vi "Day 12-1.vi"() -> ()   [LabVIEW 2020]
panel:
  out "# Paths 2":i32
  out "# Paths 1":i32
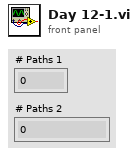
[diagram p1: front panel]
types:
  T1 = typedef "Cave System.ctl" = cluster{"Names":map{string, i32}, "Caves":T2[], "Start":i32, "End":i32}
  T2 = typedef "Cave.ctl" = cluster{"Name":string, "Index":i32, "Big":bool, "Links":i32[]}
  T3 = typedef "Path.ctl" = cluster{"Visited":bool[], "Caves":i32[]}
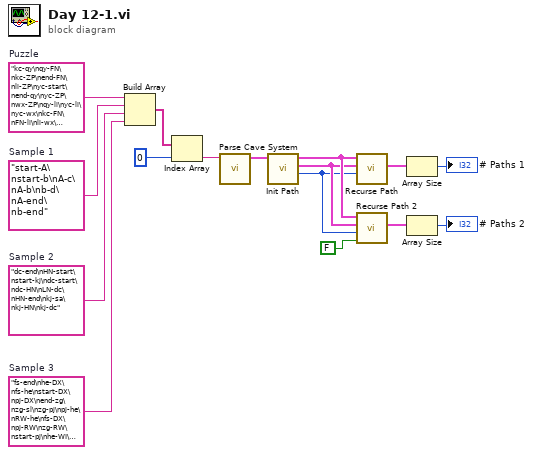
[diagram p0: block diagram]
diagram:
  w11 = "kc-qy\nqy-FN\nkc-ZP\nend-FN\nli-ZP\nyc-start\nend-qy\nyc-ZP\nwx-ZP\nqy-li\nyc-li\nyc-wx\nkc-FN\nFN-li\nli-wx\nkc-wx\nZP-start\nli-kc\nqy-nv\nZP-qy\nnv-xr\nwx-start\nend-nv\nkc-nv\nnv-XQ"  # Puzzle
  w14 = "fs-end\nhe-DX\nfs-he\nstart-DX\npj-DX\nend-zg\nzg-sl\nzg-pj\npj-he\nRW-he\nfs-DX\npj-RW\nzg-RW\nstart-pj\nhe-WI\nzg-he\npj-fs\nstart-RW"  # Sample 3
  w15 = "dc-end\nHN-start\nstart-kj\ndc-start\ndc-HN\nLN-dc\nHN-end\nkj-sa\nkj-HN\nkj-dc"  # Sample 2
  w16 = "start-A\nstart-b\nA-c\nA-b\nb-d\nA-end\nb-end"  # Sample 1
  n1 = Build Array(w11, w16, w15, w14) -> (w13:string[])
  n2 = Index Array(array=w13, index=0) -> (element=w10:string)
  n3 = call "Parse Cave System.vi"("Input"=w10) -> ("Cave System"=w9:T1)  [unwired: 10 in]
  n4 = call "Init Path.vi"("Cave System In"=w9) -> ("Start"=w4:i32, "Path"=w5:T3, "Cave System"=w6:T1)  [unwired: 8 in]
  n5 = call "Recurse Path.vi"("Next Cave"=w4, "Parent Path"=w5, "Cave System In"=w6) -> ("Found Paths"=w8:T3[])  [unwired: 8 in]
  n6 = call "Recurse Path 2.vi"("Double Visit"=FALSE, "Next Cave"=w4, "Parent Path"=w5, "Cave System In"=w6) -> ("Found Paths"=w2:T3[])  [unwired: 7 in]
  n7 = Array Size(array=w8) -> (size(s)=→"# Paths 1":i32)
  n8 = Array Size(array=w2) -> (size(s)=→"# Paths 2":i32)
